vi "S2C_ProcessStatus.vi"(8 "Error In":errorcluster) -> (0 "Error Out":errorcluster)   [LabVIEW 2015]
uses:
  Command/S2C_CMD_Globals.vi
panel:
  in  "Refresh":bool
  in  "Status":i32(listbox) caption="Process Status"
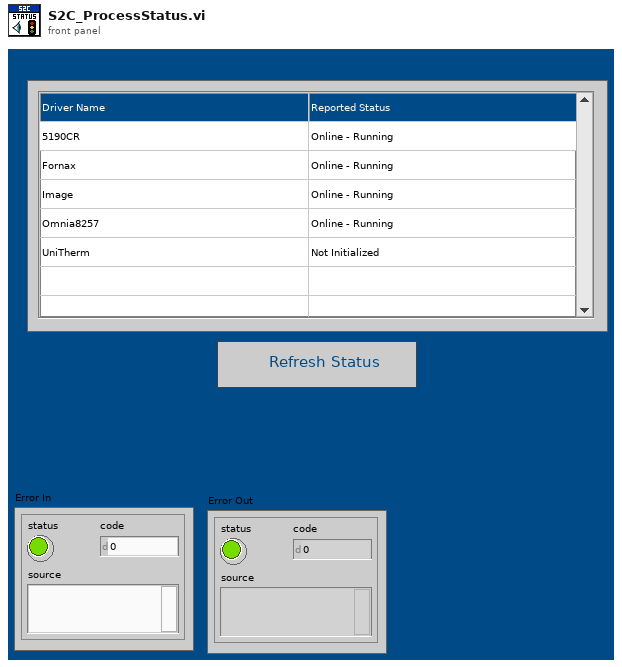
[diagram p1: front panel]
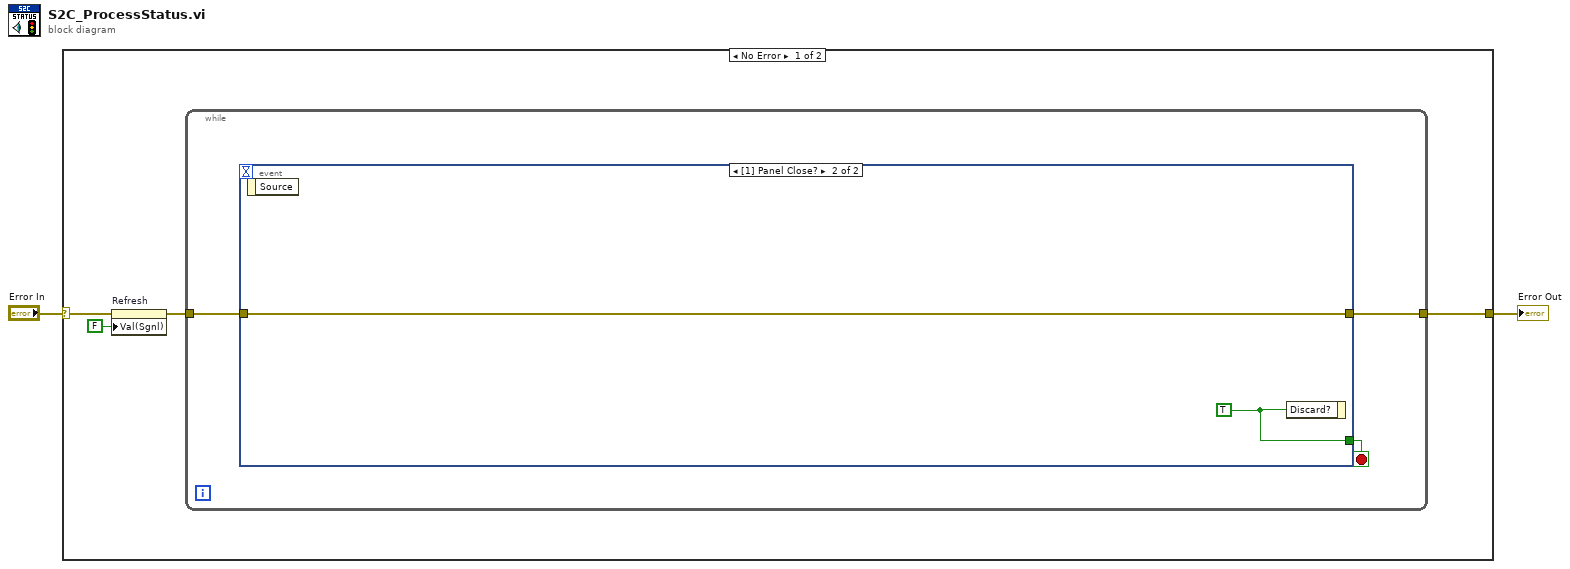
[diagram p0: block diagram]
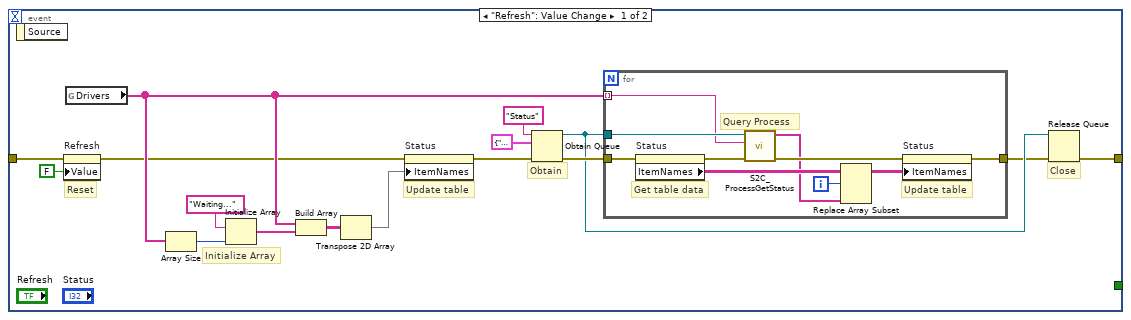
[diagram p2: hidden frame]
diagram:
  n1 = case shown="No Error" "Error In" {
    selector: "Error In" -> [w5 w38]
    tunnel: [w6 w38] -> w1
    frame No Error {
      n2 = property on="Refresh" class="Bool (strict)"(error in=w5, "Val(Sgnl)"=FALSE ("Value (Signaling)")) -> (error out=w4:errorcluster)  [unwired: 1 in, 1 out]
      n3 = while {
        tunnel: w4 -> [w9]
        tunnel: [w8] -> w6
        stop <- w7 stop-if-true
        n4 = event shown="[1] Panel Close?" {
          selector: _ -> [_ _]
          dyn-events: _ -> [_ _]
          timeout: _ -> [_ _]
          tunnel: w9 -> [w13 w37]
          tunnel: [w22 w37] -> w8
          tunnel: [_ w36] -> w7
          event "Refresh": Value Change {
            # "Reset"
            # "Update table"
            # "Initialize Array"
            # "Obtain"
            # "Close"
            n5 = event-data() -> ()  [unwired: 1 in, 1 out]
            n6 = property on="Refresh" class="Bool (strict)"(error in=w13, "Value"=FALSE ("Refresh")) -> (error out=w10:errorcluster)  [unwired: 1 in, 1 out]
            n7 = global read "S2C_CMD_Globals.vi" "Drivers"() -> (w11:string[])
            n8 = Array Size(array=w11) -> (size(s)=w17:i32)
            n9 = Initialize Array("Waiting...", w17) -> (w15:string[])
            n10 = Build Array(w11, w15) -> (w16:string[][])
            n11 = Transpose 2D Array(2D array=w16) -> (transposed array=w14:string[][])
            n12 = property on="Status" class="MCListbox (strict)"(error in=w10, "ItemNames"=w14) -> (error out=w19:errorcluster)  [unwired: 1 in, 1 out]
            n13 = Obtain Queue(name (unnamed)="Status", element data type=cluster{"Command":string, "Response":variant} {"Command"="Status", "Response"=variant} ("Request Cluster"), error in (no error)=w19) -> (queue out=w21:refnum<queue>, error out=w24:errorcluster)  [unwired: 2 in, 1 out]
            n14 = for {
              tunnel: w24 -> [w35]
              tunnel: w21 -> [w29]
              tunnel: [w31] -> w20
              tunnel: w11 -> [w28] mode=indexing
              i -> [w32]
              # "Update table"
              # "Get table data"
              # "Query Process"
              n15 = property on="Status" class="MCListbox (strict)"(error in=w35) -> (error out=w30:errorcluster, "ItemNames"=w34:string[][])  [unwired: 1 in, 1 out]
              n16 = call "S2C_ProcessGetStatus.vi"("Error In"=w30, "Driver"=w28, "Q-Ref"=w29) -> ("Error Out"=w27:errorcluster, "Response"=w26:string[])  [unwired: 7 in]
              n17 = Replace Array Subset(array=w34, new element=w26, index (row)=w32) -> (w33:string[][])  [unwired: 1 in]
              n18 = property on="Status" class="MCListbox (strict)"(error in=w27, "ItemNames"=w33) -> (error out=w31:errorcluster)  [unwired: 1 in, 1 out]
            }
            n19 = Release Queue(queue=w21, error in (no error)=w20) -> (error out=w22:errorcluster)  [unwired: 1 in, 2 out]
          }
          event Panel Close? {
            w36 = TRUE ("Discard?")
            n20 = event-data() -> ()  [unwired: 1 in, 1 out]
            n21 = event-data("Discard?"=w36) -> ()  [unwired: 1 in, 1 out]
          }
        }
      }
    }
    frame Error {
    }
  }
  "Error Out" <- w1
